vi "Horizontal Timing calculation.vi"(0 "Frequency Sweep":dbl format="%#_6p", 5 "Resolution Bandwidth(%)":dbl min=0.0 max=100.0, 7 "Sampling Rate Multiplier":dbl=2.0 min=2.0 max=100.0) -> (4 "Minimum Sampling Rate":dbl, 8 "Minimum Record Length":i32)   [LabVIEW 2020, in "LDO PSRR.lvlib"]
uses:
  LDO PSRR.lvlib
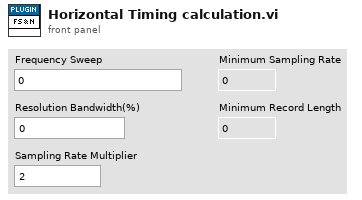
[diagram p1: front panel]
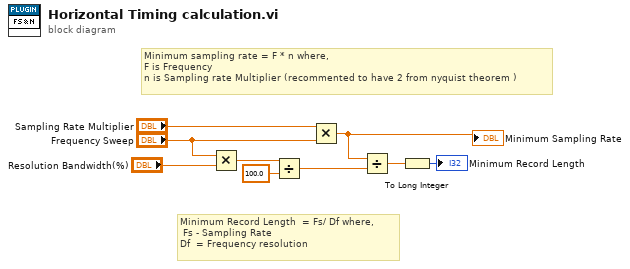
[diagram p0: block diagram]
diagram:
  # "Minimum Record Length  = Fs/ Df where,\n Fs - Sampling Rate\nDf  = Frequency resolution"
  # "Minimum sampling rate = F * n where,\nF is Frequency\nn is Sampling rate Multiplier (recommented to have 2 from nyquist theorem )"
  n1 = Multiply(x="Frequency Sweep", y="Resolution Bandwidth(%)") -> (x*y=w7:dbl)
  n2 = Divide(x=w7, y=100.0) -> (x/y=w6:dbl)
  n3 = Multiply(x="Sampling Rate Multiplier", y="Frequency Sweep") -> (x*y=w5:dbl)
  "Minimum Sampling Rate" <- w5
  n4 = Divide(x=w5, y=w6) -> (x/y=w2:dbl)
  n5 = To Long Integer(number=w2) -> (32bit integer=→"Minimum Record Length":i32)
